vi "Decode Telemetry Packet.vi"(10 "Packet Data String":string) -> (2 "Telemetry Packet":T1)   [LabVIEW 2015]
uses:
  Telemetry Packet Type.ctl
  Thermocouple Data.ctl
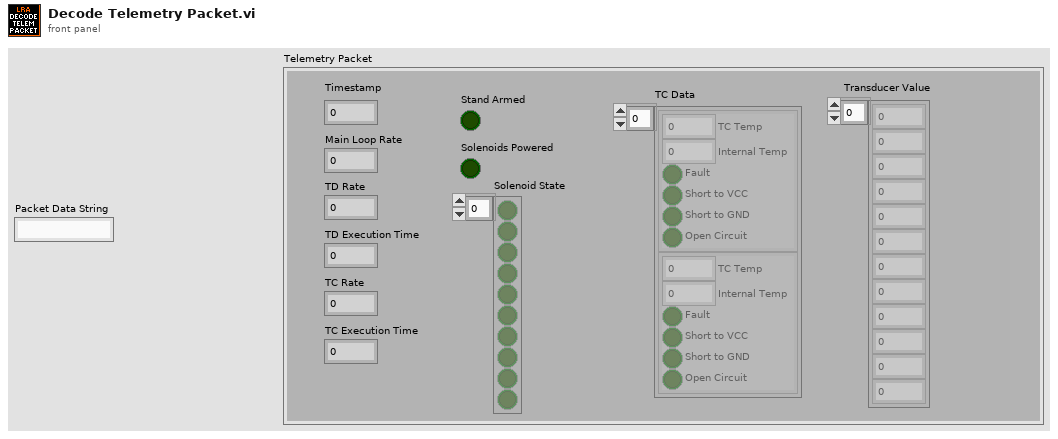
[diagram p1: front panel]
types:
  T1 = typedef "Telemetry Packet Type.ctl" = cluster{"Timestamp\n":u32, "Transducer Value":u16[], "Main Loop Rate":u32, "Solenoid State":bool[], "Stand Armed":bool, "Solenoids Powered":bool, "TC Data":T2[], "TD Rate":u32, "TD Execution Time":u32, "TC Rate":u32, "TC Execution Time":u32}
  T2 = typedef "Thermocouple Data.ctl" = cluster{"TC Temp":dbl, "Internal Temp":dbl, "Fault":bool, "Short to VCC":bool, "Short to GND":bool, "Open Circuit":bool}
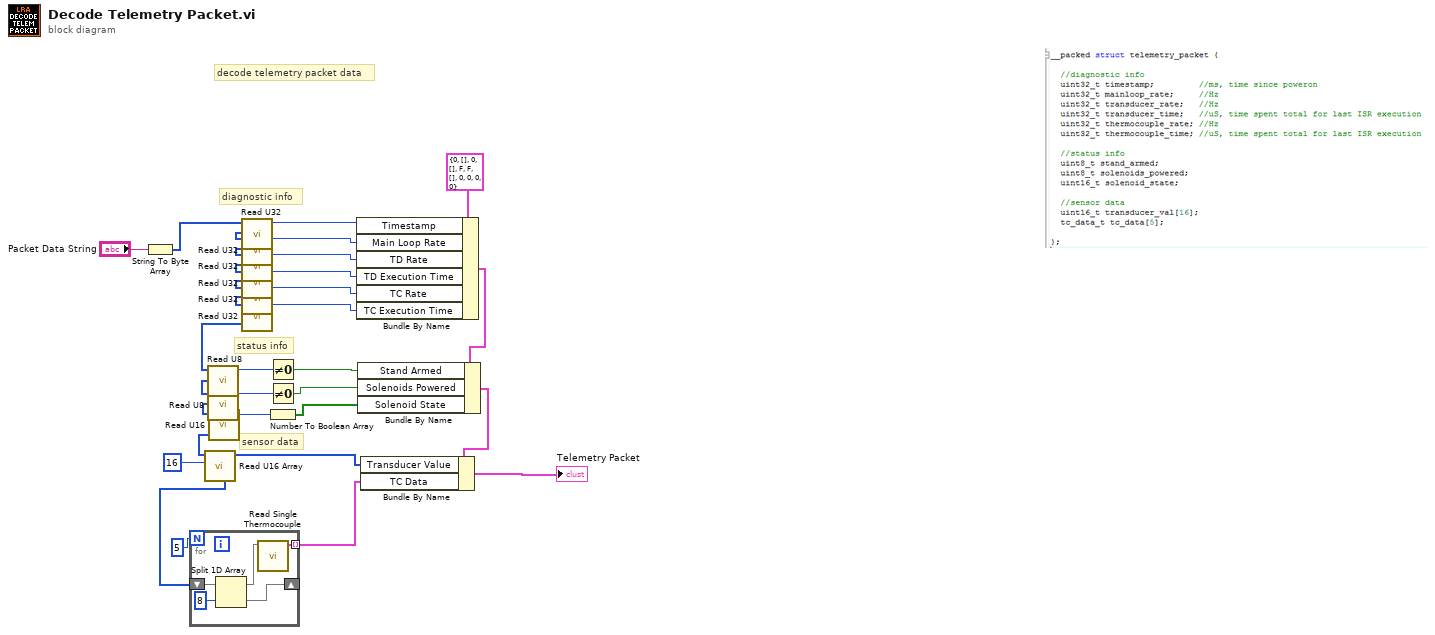
[diagram p0: block diagram]
diagram:
  # "sensor data"
  # "status info"
  # "diagnostic info"
  # "decode telemetry packet data"
  n1 = String To Byte Array(string="Packet Data String") -> (unsigned byte array=w24:u8[])
  n2 = call "Read U32.vi"("unsigned byte array"=w24) -> ("U32 Out"=w17:u32, "rest of array"=w23:u8[])  [unwired: 9 in]
  n3 = call "Read U32.vi"("unsigned byte array"=w23) -> ("U32 Out"=w16:u32, "rest of array"=w22:u8[])  [unwired: 9 in]
  n4 = call "Read U32.vi"("unsigned byte array"=w22) -> ("U32 Out"=w15:u32, "rest of array"=w21:u8[])  [unwired: 9 in]
  n5 = call "Read U32.vi"("unsigned byte array"=w21) -> ("U32 Out"=w14:u32, "rest of array"=w20:u8[])  [unwired: 9 in]
  n6 = call "Read U32.vi"("unsigned byte array"=w20) -> ("U32 Out"=w13:u32, "rest of array"=w19:u8[])  [unwired: 9 in]
  n7 = call "Read U32.vi"("unsigned byte array"=w19) -> ("U32 Out"=w12:u32, "rest of array"=w18:u8[])  [unwired: 9 in]
  n8 = call "Read U8.vi"("unsigned byte array"=w18) -> ("U8 Out"=w30:u8, "rest of array"=w26:u8[])  [unwired: 9 in]
  n9 = call "Read U8.vi"("unsigned byte array"=w26) -> ("U8 Out"=w27:u8, "rest of array"=w11:u8[])  [unwired: 9 in]
  n10 = call "Read U16.vi"("unsigned byte array"=w11) -> ("U16 Out"=w10:u16, "rest of array"=w8:u8[])  [unwired: 9 in]
  n11 = call "Read U16 Array.vi"("Size"=u32 16, "unsigned byte array"=w8) -> ("U16 Array Out"=w5:u16[], "rest of array"=w2:u8[])  [unwired: 8 in]
  n12 = for {
    N: 5 -> [_]
    shift-right: [w36] -> _
    shift-left: w2 -> [w37]
    tunnel: [w34] -> w1 mode=indexing
    n13 = Split 1D Array(array=w37, index=8) -> (first subarray=w35:u8[], second subarray=w36:u8[])
    n14 = call "Read Single Thermocouple.vi"("Packet Data"=w35) -> ("TC Data"=w34:T2)  [unwired: 10 in]
  }
  n15 = Not Equal To 0?(x=w30) -> (x != 0?=w28:bool)
  n16 = Not Equal To 0?(x=w27) -> (x != 0?=w25:bool)
  n17 = Number To Boolean Array(number=w10) -> (Boolean array=w9:bool[])
  n18 = Bundle By Name(cluster=T1 {"Timestamp\n"=0, "Transducer Value"=[], "Main Loop Rate"=0, "Solenoid State"=[], "Stand Armed"=FALSE, "Solenoids Powered"=FALSE, "TC Data"=[], "TD Rate"=0, "TD Execution Time"=0, "TC Rate"=0, "TC Execution Time"=0}, "Timestamp"=w17, "Main Loop Rate"=w16, "TD Rate"=w15, "TD Execution Time"=w14, "TC Rate"=w13, "TC Execution Time"=w12) -> (w29:T1)
  n19 = Bundle By Name(cluster=w29, "Stand Armed"=w28, "Solenoids Powered"=w25, "Solenoid State"=w9) -> (w6:T1)
  n20 = Bundle By Name(cluster=w6, "Transducer Value"=w5, "TC Data"=w1) -> (→"Telemetry Packet":T1)
